vi "Robot Main.vi"() -> ()   [LabVIEW 2019]
uses:
  Robot Global Data.vi
  <vilib>/Rock Robotics/WPI/Joystick/WPI_JoystickDeviceEnum.ctl
  DriveQuadTalonSRX/DriveQuadTalonSRX_Motor.lvlib
  <vilib>/Rock Robotics/WPI/Joystick/WPI_JoystickArcadeMapping.vi
  DriveQuadTalonSRX/Dist_Type.ctl
  DriveQuadTalonSRX/Time_Units_Control.ctl
  <vilib>/Rock Robotics/WPI/DriverStation/WPI_DriverStationRobotMode2.ctl
  MiscSupportPrograms/Radio_Speed_Ctrl.ctl
panel:
  in  "Right Speed \nDemand\nPERCENT":T1=enum."Radio Selection 7"
  in  "Left Speed \nDemand\nPERCENT":T1=enum."Radio Selection 7"
  out "VELOCITY CTRL":bool
  in  "Tab Control":enum32{"Operation", "Left Tune", "Right Tune"}(tab)
  out "Encoder Edges Per Rev":dbl=5000.0
  in  "Encoder counts Per Rev":dbl=360.0
  in  "Max Sped (Units)":dbl=20.0
  out "Robot Mode":T2
  out "LeftSpeed\nTarget":dbl format="%.2f"
  out "RigthSpeed\nTarget":dbl format="%.2f"
  in  "RIght CAN":u8=14
  in  "Left CAN":u8=13
  in  "Enable \nClosed Loop":bool=TRUE
  in  "Use \nJoyStick":bool
  out "Left Speed\nRPM":dbl format="%.2f"
  out "Right Speed\nRPM":dbl format="%.2f"
  in  "Wheel Radius In":dbl=3.0 format="%.4f"
  in  "Distance Type":T3=enum."Feet"
  in  "Time":T4
  out "Count/Dist":dbl format="%.4f"
  out "Dist/Count":dbl format="%.4f"
  out "Units":string
  out "Count/VelUnits In 0.1 SEC":dbl format="%.4f"
  out "VelUnits/Count in 0.1":dbl format="%.4f"
  in  "Gear Ratio":dbl=1.0 format="%.4f"
  in  "Left Slave CAN":u8=13
  in  "Right Slave CAN":u8=12
  in  "update left":bool
  out "Speed Closed Loop Plots RAW L":cluster{dbl, dbl}(graph)
  out "Applied Output  L":dbl format="%.5f"
  in  "Kp L":dbl=0.01611 format="%.5f"
  in  "KI L":dbl=0.0012 format="%.5f"
  in  "Kd L":dbl=0.01 format="%.5f"
  in  "FF L":dbl=0.01611 format="%.5f"
  in  "I Zone L":dbl=600.0 format="%.5f"
  out "Encoder Velocity Units Per 100ms L":dbl format="%.5f"
  out "Target Velocity Units per 100ms L":dbl format="%.5f"
  out "Motor output Plot L":cluster{"Percent Output":dbl}(graph)
  out "Raw encoder counts  L":dbl
  out "Speed Closed Loop Plots ENG L":cluster{dbl, dbl}(graph)
  out "Speed Dmd  FT/SEC L":dbl format="%.5f"
  out "Speed  FT/SEC L":dbl format="%.5f"
  in  "F Open Loop L":dbl=0.01611 format="%.5f"
  out "Distance FT L":dbl format="%.5f"
  out "Left FF\nAdj Mult":dbl format="%.6f"
  in  "update right":bool
  out "Speed Closed Loop Plots RAW R":cluster{dbl, dbl}(graph)
  out "Applied Output R":dbl format="%.5f"
  in  "Kp R":dbl=0.01611 format="%.5f"
  in  "KI R":dbl=0.0012 format="%.5f"
  in  "Kd R":dbl=0.01 format="%.5f"
  in  "FF R":dbl=0.01611 format="%.5f"
  in  "I Zone R":dbl=600.0 format="%.5f"
  out "Encoder Velocity Units Per 100ms R":dbl format="%.5f"
  out "Target Velocity Units per 100ms R":dbl format="%.5f"
  out "Motor output Plot R":cluster{"Applied Throttle":dbl}(graph)
  out "Raw encoder counts R":dbl
  out "Speed Closed Loop Plots ENG R":cluster{dbl, dbl}(graph)
  out "Speed Dmd FT/SEC R":dbl format="%.5f"
  out "Speed FT/SEC R":dbl format="%.5f"
  in  "F Open Loop R":dbl=0.01611 format="%.5f"
  out "Distance FT R":dbl format="%.5f"
  out "Right FF\nAdj Mult":dbl format="%.6f"
  # "x"
  # "Filtered\n600 ms\naverage"
  # "Set CAN ID before\nstarting execution..."
  # "original\nf .01611\np .01611\ni .0012\nd .01"
  # "original\nf .01611\np .01611\ni .0012\nd .01"
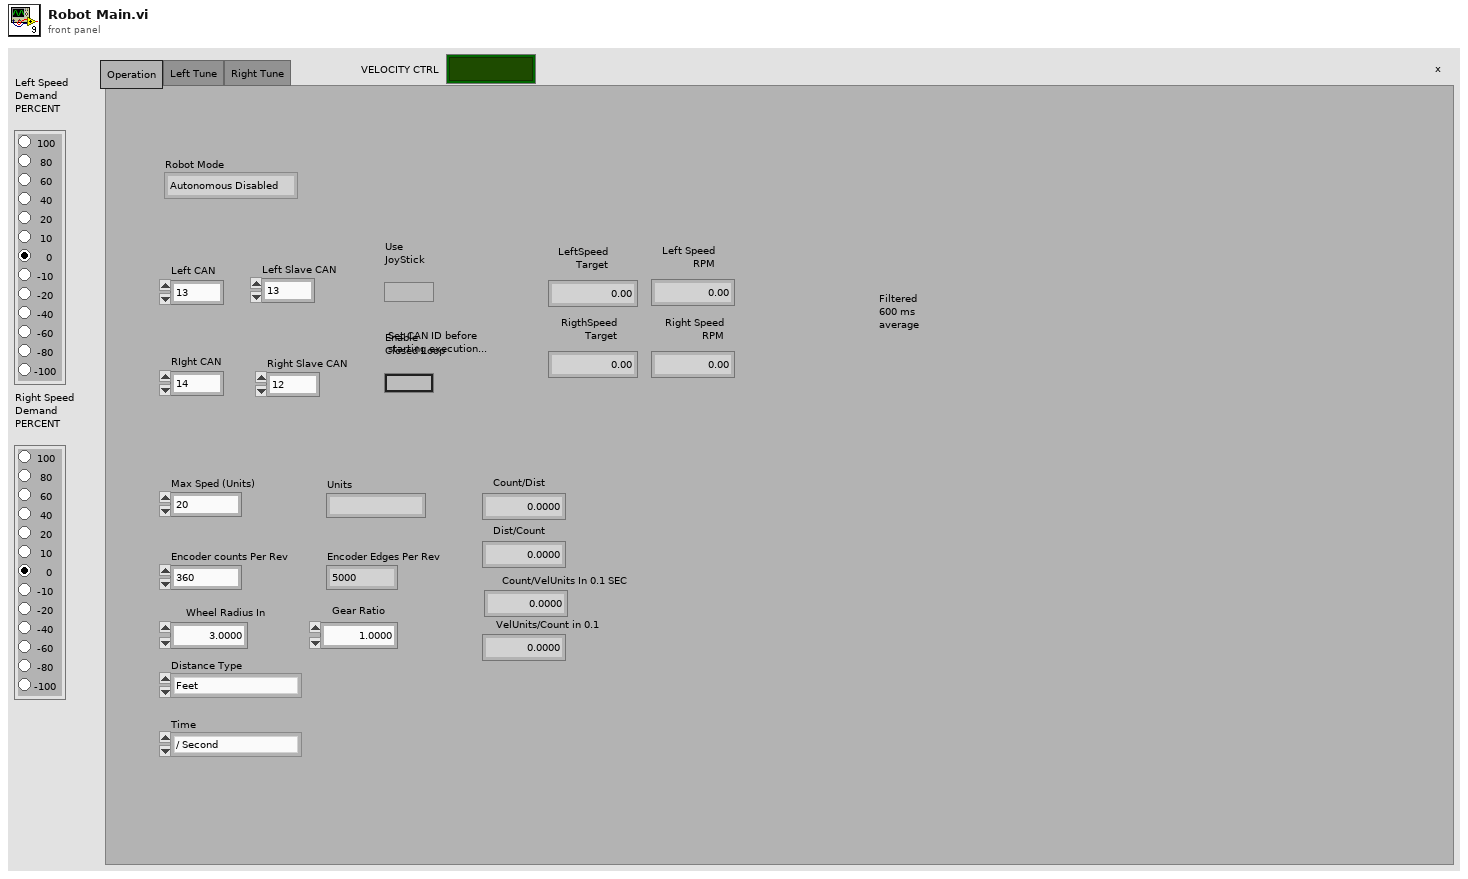
[diagram p1: front panel]
types:
  T1 = typedef "Radio_Speed_Ctrl.ctl" = enum32{"Radio Selection 1", "Radio Selection 2", "Radio Selection 3", "Radio Selection 4", "Radio Selection 5", "Radio Selection 6", "Radio Selection 7", "Radio Selection 8", "Radio Selection 9", "Radio Selection 10", "Radio Selection 11", "Radio Selection 12", "Radio Selection 13"}
  T2 = typedef "WPI_DriverStationRobotMode2.ctl" = enum16{"Autonomous Disabled", "Autonomous Enabled", "Teleop Disabled", "Teleop Enabled", "Disconnected", "Finish", "Test Disabled", "Test Enabled", "Emergency Stopped"}
  T3 = typedef "DriveQuadTalonSRX_Motor.lvlib/Dist_Type.ctl" = enum16{"Revolutions", "Feet"}
  T4 = typedef "DriveQuadTalonSRX_Motor.lvlib/Time_Units_Control.ctl" = enum16{"/ Second", "/ Minute"}
  T5 = typedef "WPI_JoystickDeviceEnum.ctl" = enum16{"USB 0", "USB 1", "USB 2", "USB 3", "USB 4", "USB 5"}
  T6 = typedef "WPI_JoystickDevRef.ctl" = cluster{"Device":T5}
  T7 = typedef "DriveQuadTalonSRX_Motor.lvlib/ctrlRef_DriveQuadTalon.ctl" = cluster{"LeftMasterDriveRef":T8, "RightMasterDriveRef":T8}
  T8 = typedef "WPI_MotorControlDeviceRef.ctl" = cluster{"DeviceStatus":errorcluster, "Type":T9, "PWM":cluster{"PWM Channel":T10, "DeadBand":T11}, "CAN":cluster{"Device Number":u8, "SetOutput VI Ref":variant, "GetOutput VI Ref":variant, "Enable VI Ref":variant, "Disable VI Ref":variant, "Data":variant}, "Invert":bool, "DIO PWM":cluster{"PWM \"Enable\" Channel":T10, "DIOChannel":T12, "PWM Rate":dbl}}
  T9 = typedef "WPI_MotorControlType.ctl" = enum16{"PWM", "CAN", "DIO PWM"}
  T10 = typedef "FPGA_DIOPWMChannel.ctl" = enum8{"PWM 0", "PWM 1", "PWM 2", "PWM 3", "PWM 4", "PWM 5", "PWM 6", "PWM 7", "PWM 8", "PWM 9", "PWM MXP 0", "PWM MXP 1", "PWM MXP 2", "PWM MXP 3", "PWM MXP 4", "PWM MXP 5", "PWM MXP 6", "PWM MXP 7", "PWM MXP 8", "PWM MXP 9", "Invalid"}
  T11 = typedef "WPI_PWMDeadband.ctl" = cluster{"Name":string, "maxPositivePwm":i32, "minPositivePwm":i32, "centerPwm":i32, "maxNegativePwm":i32, "minNegativePwm":i32, "angularRange":u16}
  T12 = typedef "FPGA_DIOChannel.ctl" = enum8{"DIO 0", "DIO 1", "DIO 2", "DIO 3", "DIO 4", "DIO 5", "DIO 6", "DIO 7", "DIO 8", "DIO 9", "DIO MXP 0", "DIO MXP 1", "DIO MXP 2", "DIO MXP 3", "DIO MXP 4", "DIO MXP 5", "DIO MXP 6", "DIO MXP 7", "DIO MXP 8", "DIO MXP 9", "DIO MXP 10", "DIO MXP 11", "DIO MXP 12", "DIO MXP 13", "DIO MXP 14", "DIO MXP 15", "SPI Port CS1", "SPI Port CS2", "SPI Port CS3", "SPI Port MISO", "SPI Port MOSI", "Invalid"}
  T13 = cluster{"Speed Dmd  FT/SEC L":dbl, "Speed  FT/SEC L":dbl}
  T14 = cluster{"Target Velocity Units per 100ms L":dbl, "Encoder Velocity Units Per 100ms L":dbl}
  T15 = cluster{"Target Velocity Units in 100ms R":dbl, "Encoder Velocity Units in 100ms R":dbl}
  T16 = cluster{"Speed Dmd FT/SEC R":dbl, "Speed FT/SEC R":dbl}
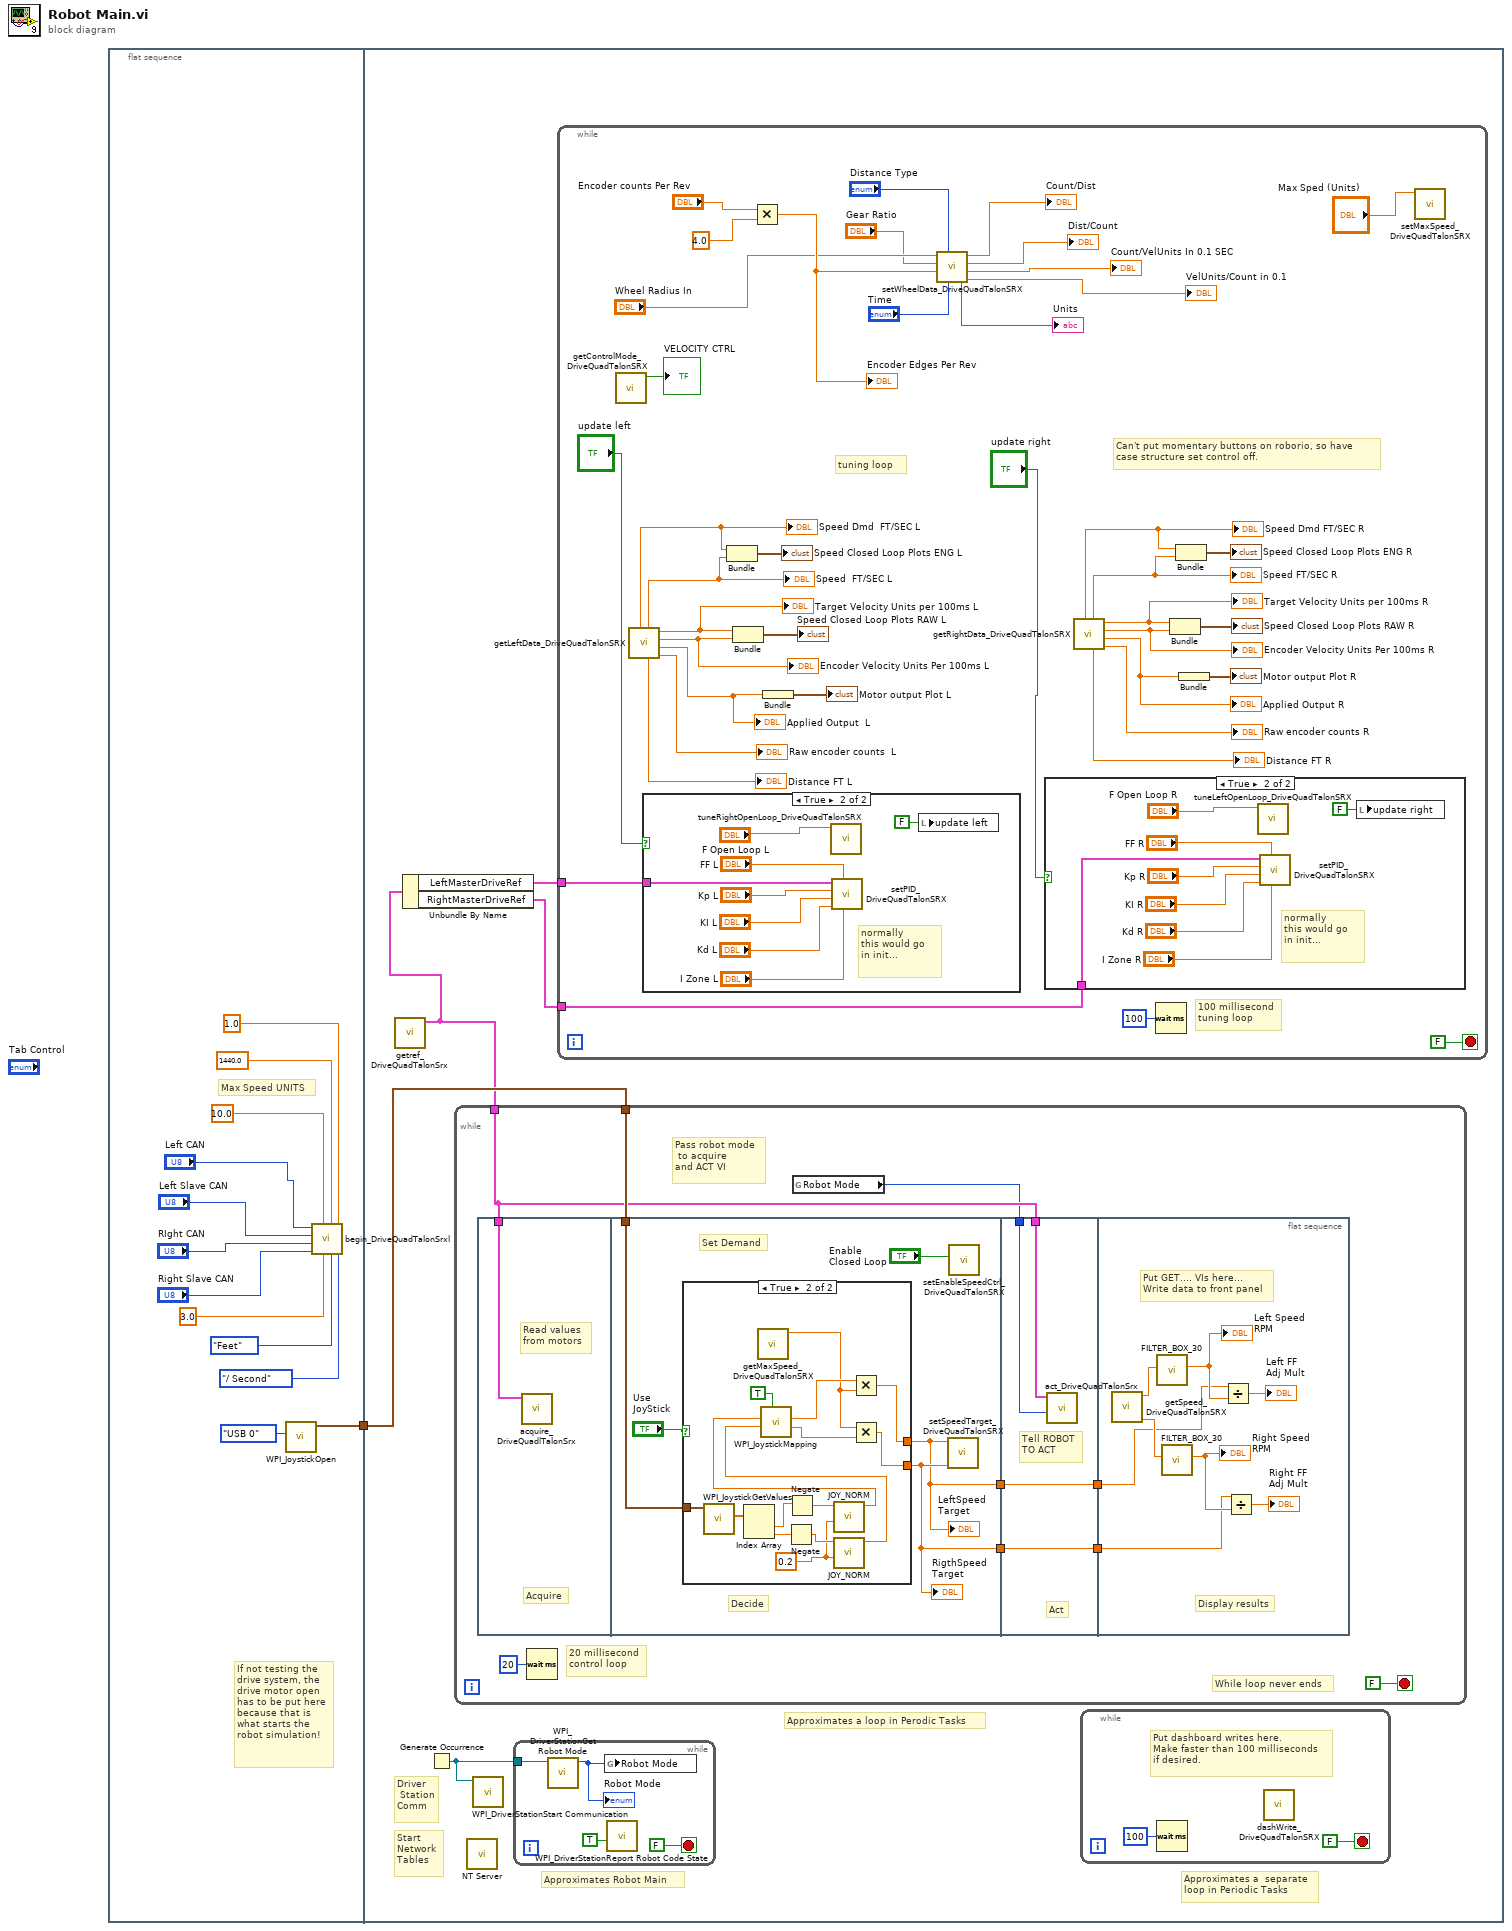
[diagram p0: block diagram]
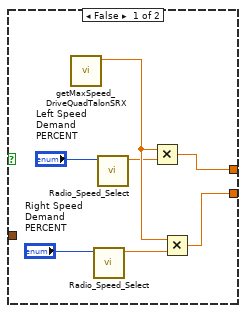
[diagram p4: hidden frame]
diagram:
  n1 = flat-sequence {
    tunnel: [w12] -> w1
    tunnel: w1 -> [w17]
    frame #0 {
      # "Max Speed UNITS"
      # "If not testing the\ndrive system, the\ndrive motor open\nhas to be put here\nbecause that is \nwhat starts the\nrobot simulation!"
      n2 = call <vilib>:"WPI_JoystickOpen.vi"("JoystickDevice"=WPI_JoystickDeviceEnum."USB 0") -> ("JoystickDevRef"=w12:T6)  [unwired: 10 in]
      n3 = call "begin_DriveQuadTalonSrxl.vi"("Time"=Time_Units_Control."/ Second", "Gear Ratio"=1.0, "Distance Type"=Dist_Type."Feet", "Enc Edges / Rev"=1440.0, "Wheel Radius In"=3.0, "MAX DESIRED\nVELOCITY\n(UNITS)"=10.0 ("MAX DESIRED\nVELOCITY\n(UNITS)"), "Right Slave CAN"="Right Slave CAN", "RIght Master CAN"="RIght CAN", "Left Slave CAN"="Left Slave CAN", "Left Master CAN"="Left CAN") -> ()  [unwired: 2 in]
    }
    frame #1 {
      # "Approximates a  separate\nloop in Periodic Tasks"
      # "Approximates a loop in Perodic Tasks"
      # "Approximates Robot Main"
      # "Start\nNetwork\nTables"
      # "Driver\n Station\nComm"
      n4 = call "getref_DriveQuadTalonSrx.vi"() -> ("DriveRef"=w16:T7)  [unwired: 11 in]
      n5 = Unbundle By Name(w16) -> ("LeftMasterDriveRef"=w15:T8, "RightMasterDriveRef"=w14:T8)
      n6 = Generate Occurrence() -> (w18:refnum<k4>)
      n7 = while {
        tunnel: w17 -> [w87]
        tunnel: w16 -> [w86]
        stop <- FALSE stop-if-true
        # "While loop never ends"
        # "Pass robot mode\n to acquire\nand ACT VI"
        # "20 millisecond\ncontrol loop"
        n8 = flat-sequence {
          tunnel: w86 -> [w90]
          tunnel: w87 -> [w95]
          tunnel: [w92] -> w83
          tunnel: [w91] -> w81
          tunnel: w86 -> [w121]
          tunnel: w85 -> [w120]
          tunnel: [w119] -> w84
          tunnel: w83 -> [w119]
          tunnel: [w118] -> w82
          tunnel: w81 -> [w118]
          tunnel: w84 -> [w125]
          tunnel: w82 -> [w124]
          frame #0 {
            # "Read values\nfrom motors"
            # "Acquire"
            n9 = call "acquire_DriveQuadlTalonSrx.vi"("QuadTalonSRXDriveRef"=w90) -> ()  [unwired: 10 in, 1 out]
          }
          frame #1 {
            # "Set Demand"
            # "Decide"
            n10 = case shown="True" "Use \nJoyStick" {
              tunnel: w95 -> [_ w112]
              tunnel: [w97 w109] -> w91
              tunnel: [w96 w111] -> w92
              frame False {
                n11 = call "getMaxSpeed_DriveQuadTalonSRX.vi"() -> ("Max Speed"=w100:dbl)  [unwired: 9 in, 1 out]
                n12 = call "Radio_Speed_Select.vi"("Left Speed \nDemand\nPERCENT"="Right Speed \nDemand\nPERCENT") -> ("PERCENT"=w98:dbl)  [unwired: 10 in]
                n13 = call "Radio_Speed_Select.vi"("Left Speed \nDemand\nPERCENT"="Left Speed \nDemand\nPERCENT") -> ("PERCENT"=w99:dbl)  [unwired: 10 in]
                n14 = Multiply(x=w100, y=w99) -> (x*y=w97:dbl)
                n15 = Multiply(x=w100, y=w98) -> (x*y=w96:dbl)
              }
              frame True {
                w106 = 0.2 ("Deadband")
                n16 = call <vilib>:"WPI_JoystickGetValues.vi"("JoystickDevRef"=w112) -> ("Axes"=w117:dbl[])  [unwired: 6 in, 4 out]
                n17 = Index Array(array=w117) -> (element #1=w115:dbl, element #2=w116:dbl)  [unwired: 2 in]
                n18 = call "getMaxSpeed_DriveQuadTalonSRX.vi"() -> ("Max Speed"=w103:dbl)  [unwired: 9 in, 1 out]
                n19 = Negate(x=w116) -> (-x=w107:dbl)
                n20 = Negate(x=w115) -> (-x=w108:dbl)
                n21 = call "JOY_NORM.vi"("Deadband"=w106, "Joy Input"=w108) -> ("Joy Output"=w105:dbl)  [unwired: 9 in]
                n22 = call "JOY_NORM.vi"("Deadband"=w106, "Joy Input"=w107) -> ("Joy Output"=w104:dbl)  [unwired: 9 in]
                n23 = call-poly <vilib>:"WPI_JoystickMapping.vi"("Square Inputs"=TRUE, "Y axis value"=w104, "X axis value"=w105) -> ("Right Motor Value"=w110:dbl, "Left Motor Value"=w113:dbl)  [unwired: 7 in]
                n24 = Multiply(x=w113, y=w103) -> (x*y=w109:dbl)
                n25 = Multiply(x=w103, y=w110) -> (x*y=w111:dbl)
              }
            }
            "RigthSpeed\nTarget" <- w92
            "LeftSpeed\nTarget" <- w91
            n26 = call "setSpeedTarget_DriveQuadTalonSRX.vi"("Right Speed Target\nFt/SEC"=w92, "Left Speed Target\nFT/SEC"=w91) -> ()  [unwired: 9 in]
            n27 = call "setEnableSpeedCtrl_DriveQuadTalonSRX.vi"("Enable Speed Control"="Enable \nClosed Loop") -> ()  [unwired: 10 in]
          }
          frame #2 {
            # "Tell ROBOT\nTO ACT"
            # "Act"
            n28 = call "act_DriveQuadTalonSrx.vi"("Robot Mode"=w120, "QuadTalonSRXDriveRef"=w121) -> ()  [unwired: 9 in, 1 out]
          }
          frame #3 {
            # "Put GET.... VIs here...  \nWrite data to front panel"
            # "Display results"
            n29 = call "getSpeed_DriveQuadTalonSRX.vi"() -> ("Right Speed Ft/SEC"=w128:dbl, "Left Speed FT/SEC"=w129:dbl)  [unwired: 9 in]
            n30 = call "FILTER_BOX_30.vi"("Input"=w129) -> ("Filtered_Value"=w127:dbl)  [unwired: 10 in]
            "Left Speed\nRPM" <- w127
            n31 = call "FILTER_BOX_30.vi"("Input"=w128) -> ("Filtered_Value"=w126:dbl)  [unwired: 10 in]
            "Right Speed\nRPM" <- w126
            n32 = Divide(x=w124, y=w127) -> (x/y=→"Left FF\nAdj Mult":dbl)
            n33 = Divide(x=w125, y=w126) -> (x/y=→"Right FF\nAdj Mult":dbl)
          }
        }
        n34 = Wait (ms)(milliseconds to wait=u32 20) -> ()  [unwired: 1 out]
        n35 = global read "Robot Global Data.vi" "Robot Mode"() -> (w85:T2)
      }
      n36 = call <vilib>:"NT Server.vi"() -> ()  [unwired: 12 in]
      n37 = call <vilib>:"WPI_DriverStationStart Communication.vi"("occurrence"=w18) -> ()  [unwired: 11 in]
      n38 = while {
        tunnel: w18 -> [w80]
        stop <- FALSE stop-if-true
        n39 = call <vilib>:"WPI_DriverStationGet Robot Mode.vi"("DS Occurrence"=w80) -> ("Robot Mode"=w77:T2)  [unwired: 1 in, 9 out]
        "Robot Mode" <- w77
        n40 = global write "Robot Global Data.vi" "Robot Mode"(w77) -> ()
        n41 = call <vilib>:"WPI_DriverStationReport Robot Code State.vi"("TeleOp"=TRUE ("Autonomous")) -> ()  [unwired: 10 in, 1 out]
      }
      n42 = while {
        tunnel: w15 -> [w56]
        tunnel: w14 -> [w55]
        stop <- FALSE stop-if-true
        # "Can't put momentary buttons on roborio, so have\ncase structure set control off."
        # "tuning loop"
        # "100 millisecond\ntuning loop"
        n43 = call "getControlMode_DriveQuadTalonSRX.vi"() -> ("VELOCITY CTRL"=→"VELOCITY CTRL":bool)  [unwired: 11 in]
        n44 = call "getLeftData_DriveQuadTalonSRX.vi"() -> ("Raw encoder counts  L"=→"Raw encoder counts  L":dbl, "Applied Output  L"=w47:dbl, "Encoder Velocity Units Per 100ms L"=w48:dbl, "Target Velocity Units per 100ms L"=w49:dbl, "Distance FT L"=→"Distance FT L":dbl, "Speed  FT/SEC L"=w50:dbl, "Speed Dmd  FT/SEC L"=w44:dbl)  [unwired: 5 in]
        "Applied Output  L" <- w47
        "Encoder Velocity Units Per 100ms L" <- w48
        "Target Velocity Units per 100ms L" <- w49
        "Speed Dmd  FT/SEC L" <- w44
        "Speed  FT/SEC L" <- w50
        n45 = case shown="True" "update left" {
          tunnel: w56 -> [_ w74]
          frame False {
          }
          frame True {
            # "normally\nthis would go\nin init..."
            n46 = call "tuneRightOpenLoop_DriveQuadTalonSRX.vi"("F Open Loop L"="F Open Loop L") -> ()  [unwired: 11 in]
            n47 = call "setPID_DriveQuadTalonSRX.vi"("I ZONE"="I Zone L", "FF"="FF L", "KD"="Kd L", "KI"="KI L", "KP"="Kp L", "MasterDriveRef"=w74) -> ()  [unwired: 6 in]
            n48 = local write "update left"(FALSE ("update left")) -> ()
          }
        }
        n49 = Bundle("Speed Dmd  FT/SEC L"=w44, "Speed  FT/SEC L"=w50) -> (→"Speed Closed Loop Plots ENG L":T13)  [unwired: 1 in]
        n50 = Bundle("Target Velocity Units per 100ms L"=w49, "Encoder Velocity Units Per 100ms L"=w48) -> (→"Speed Closed Loop Plots RAW L":T14)  [unwired: 1 in]
        n51 = Multiply(x="Encoder counts Per Rev", y=4.0) -> (x*y=w28:dbl)
        "Encoder Edges Per Rev" <- w28
        n52 = Bundle("Applied Output  L"=w47) -> (→"Motor output Plot L":cluster{"Applied Output  L":dbl})  [unwired: 1 in]
        n53 = call "setWheelData_DriveQuadTalonSRX.vi"("Time"="Time", "Distance Type"="Distance Type", "Enc Edges / Rev"=w28, "Gear Ratio"="Gear Ratio", "Wheel Radius In"="Wheel Radius In") -> ("VelUnits/Count in 0.1"=→"VelUnits/Count in 0.1":dbl, "Count/VelUnits In 0.1 SEC"=→"Count/VelUnits In 0.1 SEC":dbl, "Dist/Count"=→"Dist/Count":dbl, "Count/Dist"=→"Count/Dist":dbl, "Units"=→"Units":string)  [unwired: 2 in]
        n54 = case shown="True" "update right" {
          tunnel: w55 -> [_ w66]
          frame False {
          }
          frame True {
            # "normally\nthis would go\nin init..."
            n55 = call "tuneLeftOpenLoop_DriveQuadTalonSRX.vi"("F Open Loop R"="F Open Loop R") -> ()  [unwired: 11 in]
            n56 = call "setPID_DriveQuadTalonSRX.vi"("I ZONE"="I Zone R", "FF"="FF R", "KD"="Kd R", "KI"="KI R", "KP"="Kp R", "MasterDriveRef"=w66) -> ()  [unwired: 6 in]
            n57 = local write "update right"(FALSE ("update right")) -> ()
          }
        }
        n58 = call "getRightData_DriveQuadTalonSRX.vi"() -> ("Raw encoder counts R"=→"Raw encoder counts R":dbl, "Applied Output R"=w36:dbl, "Encoder Velocity Units in 100ms R"=w38:dbl, "Target Velocity Units in 100ms R"=w39:dbl, "Distance FT R"=→"Distance FT R":dbl, "Speed FT/SEC R"=w34:dbl, "Speed Dmd FT/SEC R"=w33:dbl)  [unwired: 5 in]
        "Applied Output R" <- w36
        "Encoder Velocity Units Per 100ms R" <- w38
        "Target Velocity Units per 100ms R" <- w39
        "Speed Dmd FT/SEC R" <- w33
        "Speed FT/SEC R" <- w34
        n59 = Wait (ms)(milliseconds to wait=u32 100) -> ()  [unwired: 1 out]
        n60 = Bundle("Target Velocity Units in 100ms R"=w39, "Encoder Velocity Units in 100ms R"=w38) -> (→"Speed Closed Loop Plots RAW R":T15)  [unwired: 1 in]
        n61 = Bundle("Speed Dmd FT/SEC R"=w33, "Speed FT/SEC R"=w34) -> (→"Speed Closed Loop Plots ENG R":T16)  [unwired: 1 in]
        n62 = Bundle("Applied Output R"=w36) -> (→"Motor output Plot R":cluster{"Applied Output R":dbl})  [unwired: 1 in]
        n63 = call "setMaxSpeed_DriveQuadTalonSRX.vi"("MAX DESIRED\nVELOCITY (UNITS)"="Max Sped (Units)") -> ()  [unwired: 8 in, 2 out]
      }
      n64 = while {
        stop <- FALSE stop-if-true
        # "Put dashboard writes here.\nMake faster than 100 milliseconds\nif desired."
        n65 = Wait (ms)(milliseconds to wait=u32 100) -> ()  [unwired: 1 out]
        n66 = call "dashWrite_DriveQuadTalonSRX.vi"() -> ()  [unwired: 12 in]
      }
    }
  }
